vi "subvi_calculate_sizes.vi"(0 "Metadata":T7, 1 "font settings":T5={"Font Name:"="Arial", "Size"=12, "Strikeout?"=FALSE, "Italic?"=FALSE, "Underline?"=FALSE, "Outline?"=FALSE, "Shadow?"=FALSE, "Bold?"=FALSE}, 2 "Color settings":T6={"Background color"=0, "Information color"=16777215}, 3 "Spacing":T3, 4 "loaded picture":picture) -> (5 "modified pictures":picture)   [LabVIEW 2016]
uses:
  cluster_metadata.ctl
  cluster_colorsettings.ctl
  cluster_spacing.ctl
  cluster_background.ctl
panel:
  in  "Dimensions":T1
  in  "Coordinates":T2
  # "x and y are the distance between the\nlower left corner of the background box and the\nlower left corner of the bar"
  # "x and y are the distance between the\nlower left corner of the image and the\nlower left corner of the box"
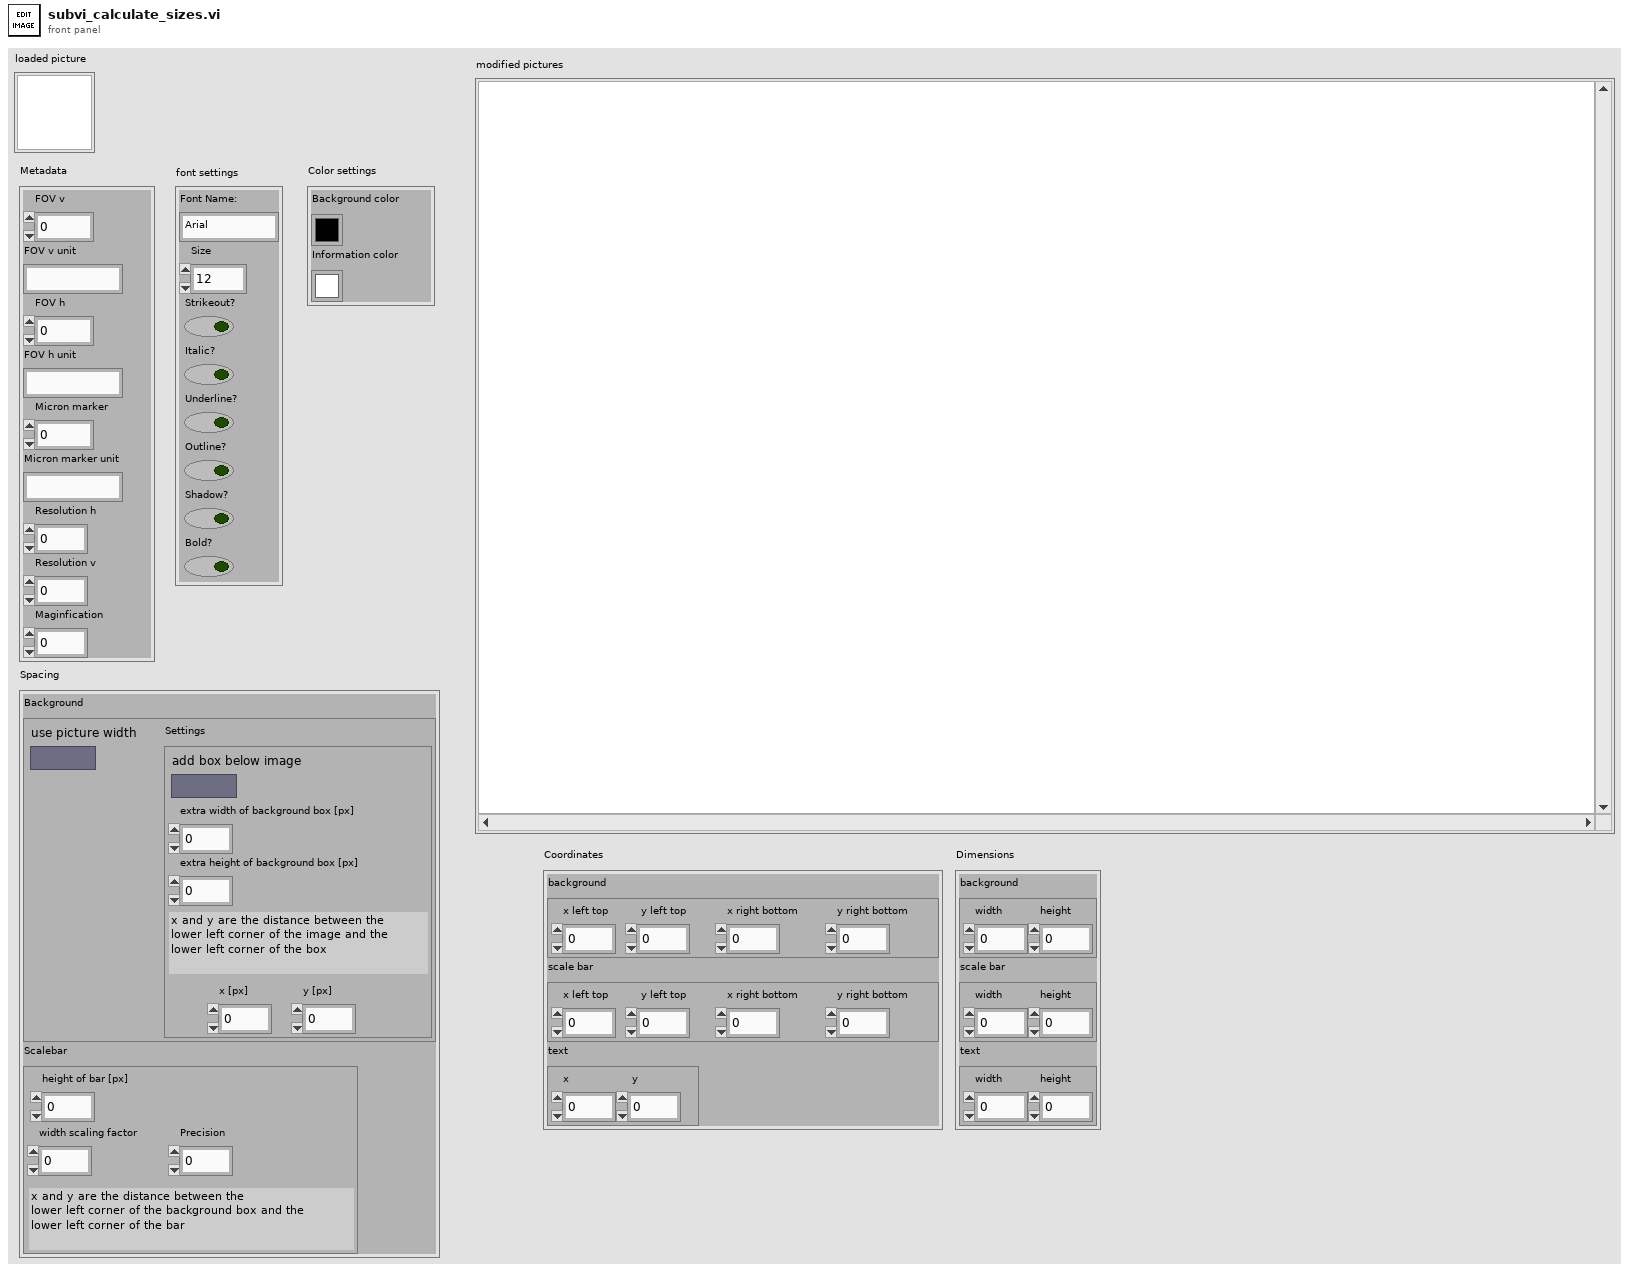
[diagram p1: front panel]
types:
  T1 = cluster{"background":cluster{"width":dbl, "height":dbl}, "scale bar":cluster{"width":dbl, "height":dbl}, "text":cluster{"width":dbl, "height":dbl}}
  T2 = cluster{"background":cluster{"x left top":dbl, "y left top":dbl, "x right bottom":dbl, "y right bottom":dbl}, "scale bar":cluster{"x left top":dbl, "y left top":dbl, "x right bottom":dbl, "y right bottom":dbl}, "text":cluster{"x ":dbl, "y":dbl}}
  T3 = typedef "cluster_spacing.ctl" = cluster{"Background":T4, "Scalebar":cluster{"height of bar [px]":dbl, "width scaling factor":dbl, "Precision":i16}}
  T4 = typedef "cluster_background.ctl" = cluster{"use picture width":bool, "Settings":cluster{"add box below image":bool, "extra width background":i16, "extra height background":i16, "x [px]":dbl, "y [px]":dbl}}
  T5 = cluster{"Font Name:":string, "Size":i16, "Strikeout?":bool, "Italic?":bool, "Underline?":bool, "Outline?":bool, "Shadow?":bool, "Bold?":bool}
  T6 = typedef "cluster_colorsettings.ctl" = cluster{"Background color":u32, "Information color":u32}
  T7 = typedef "cluster_metadata.ctl" = cluster{"FOV v":dbl, "FOV v unit":string, "FOV h":dbl, "FOV h unit":string, "Micron marker":dbl, "Micron marker unit":string, "Resolution h":i32, "Resolution v":i32, "Maginfication":i32}
  T8 = cluster{"horizontal":enum16{"left", "center", "right"}, "vertical":enum16{"top", "center", "bottom"}}
  T9 = enum16{"User-specified Font", "Application Font", "System Font", "Dialog Font"}
  T10 = cluster{"left":i16, "top":i16, "right":i16, "bottom":i16}
  T11 = cluster{"x left top":dbl, "y left top":dbl, "x right bottom":dbl, "y right bottom":dbl}
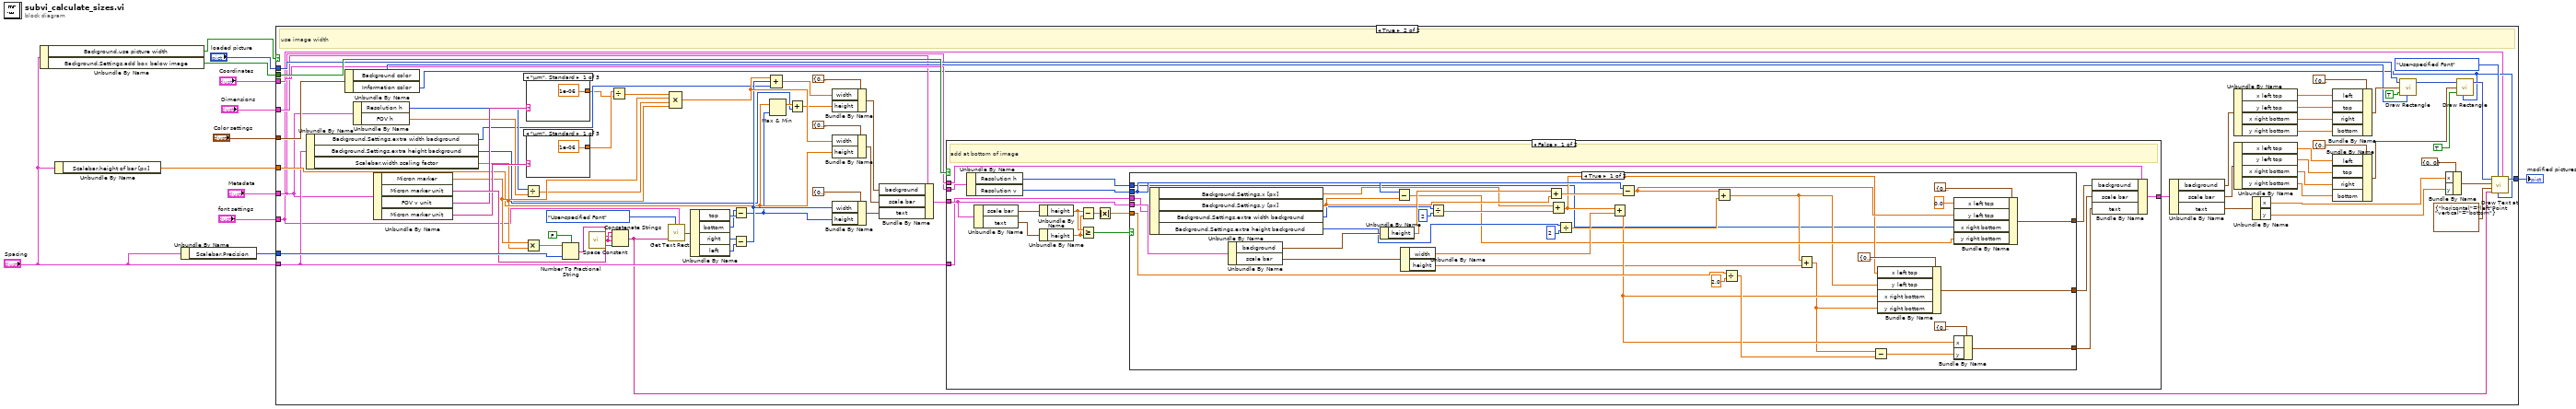
[diagram p0: block diagram]
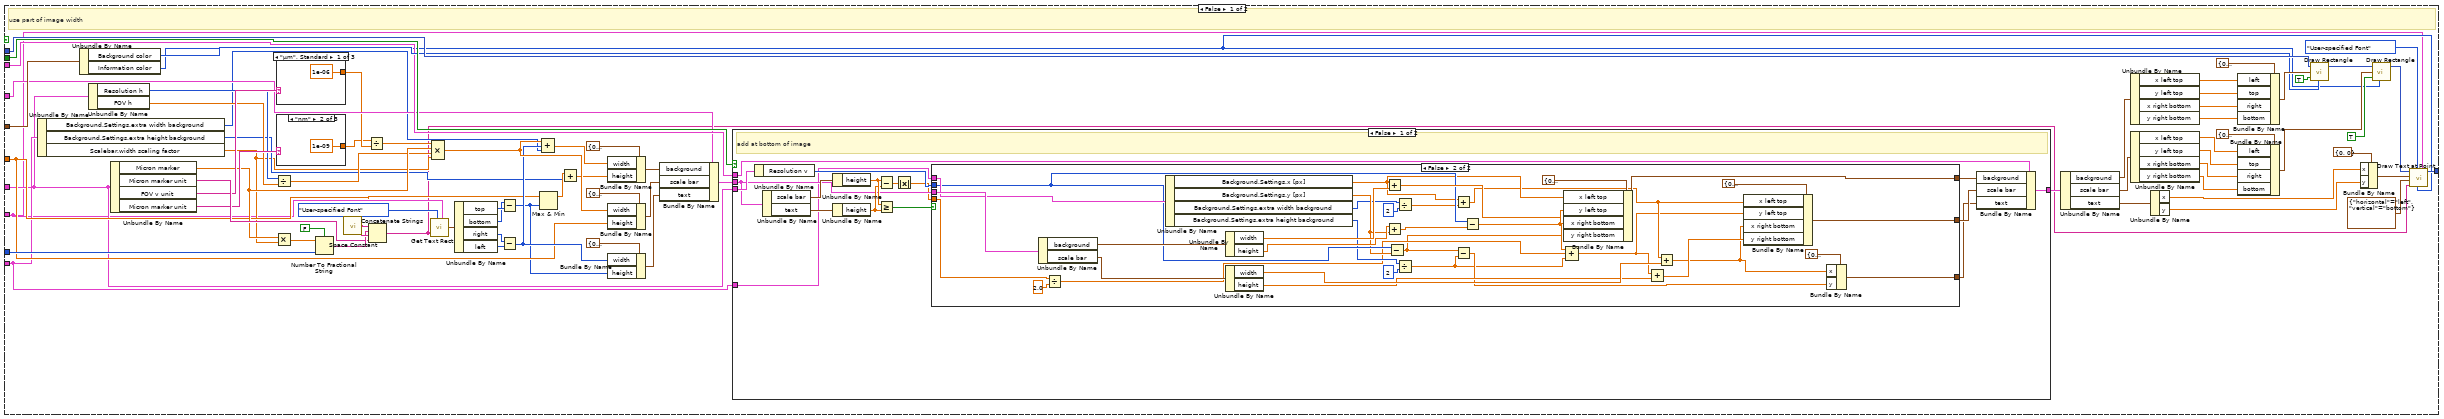
[diagram p2: hidden frame]
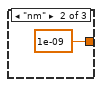
[diagram p3: hidden frame]
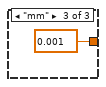
[diagram p4: hidden frame]
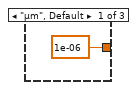
[diagram p5: hidden frame]
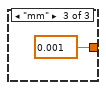
[diagram p6: hidden frame]
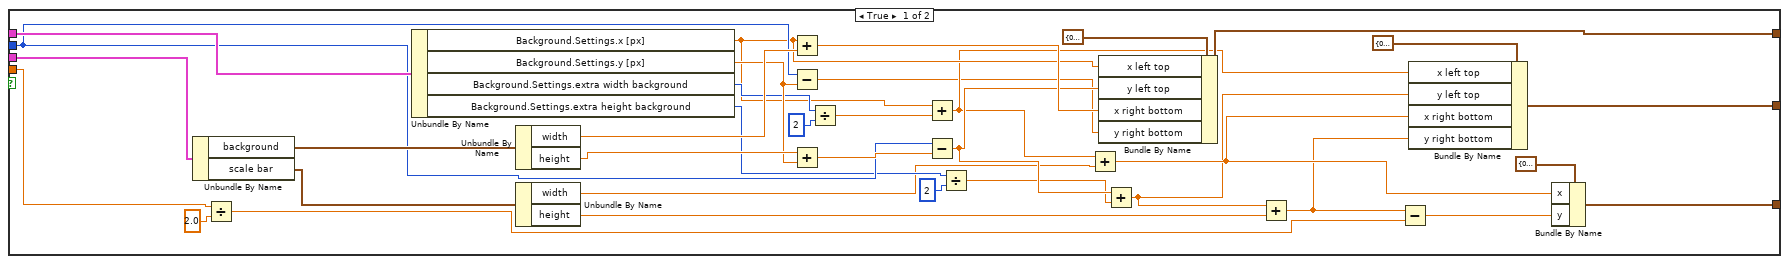
[diagram p7: hidden frame]
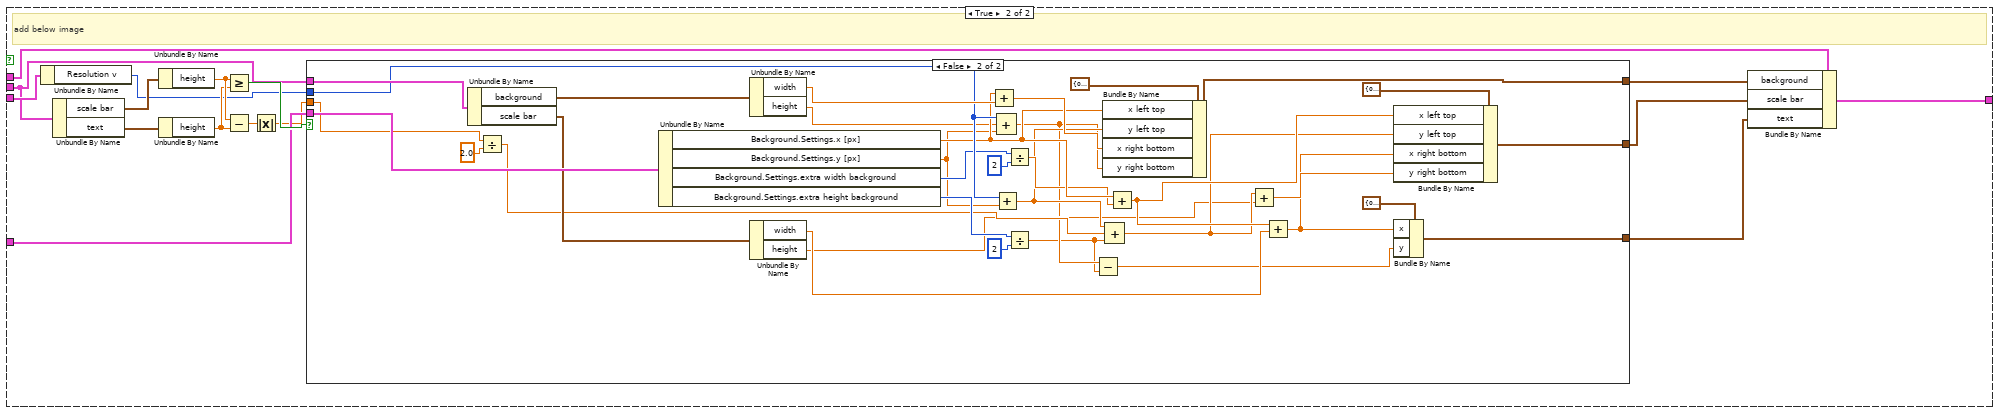
[diagram p8: hidden frame]
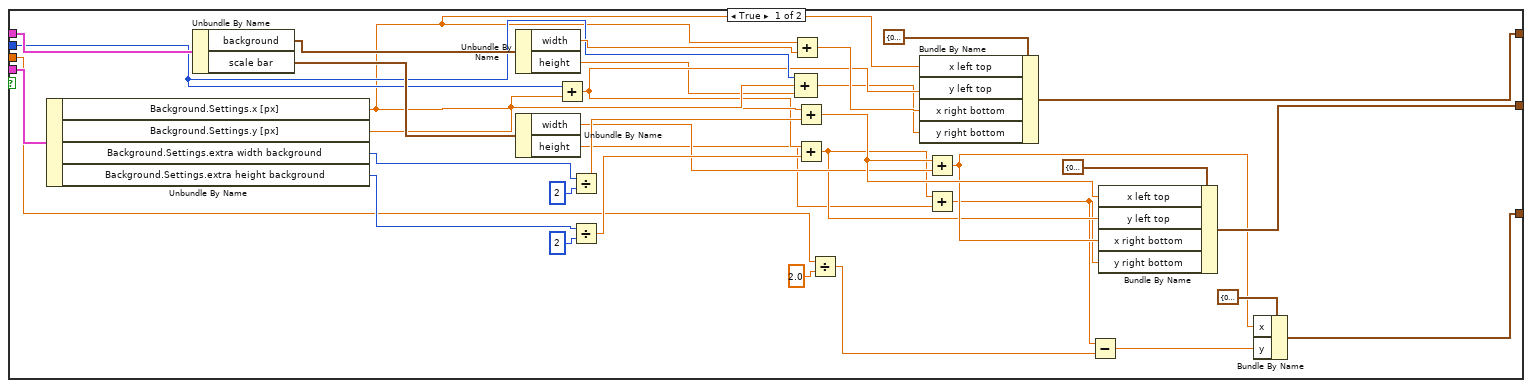
[diagram p9: hidden frame]
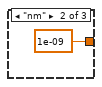
[diagram p10: hidden frame]
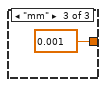
[diagram p11: hidden frame]
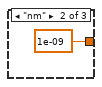
[diagram p12: hidden frame]
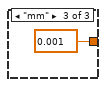
[diagram p13: hidden frame]
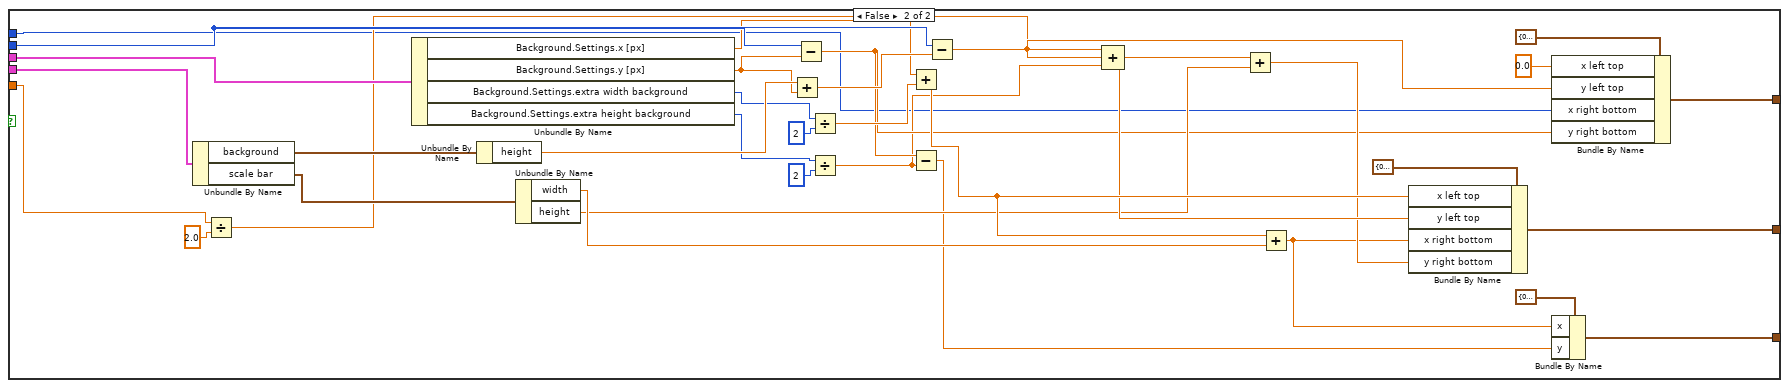
[diagram p14: hidden frame]
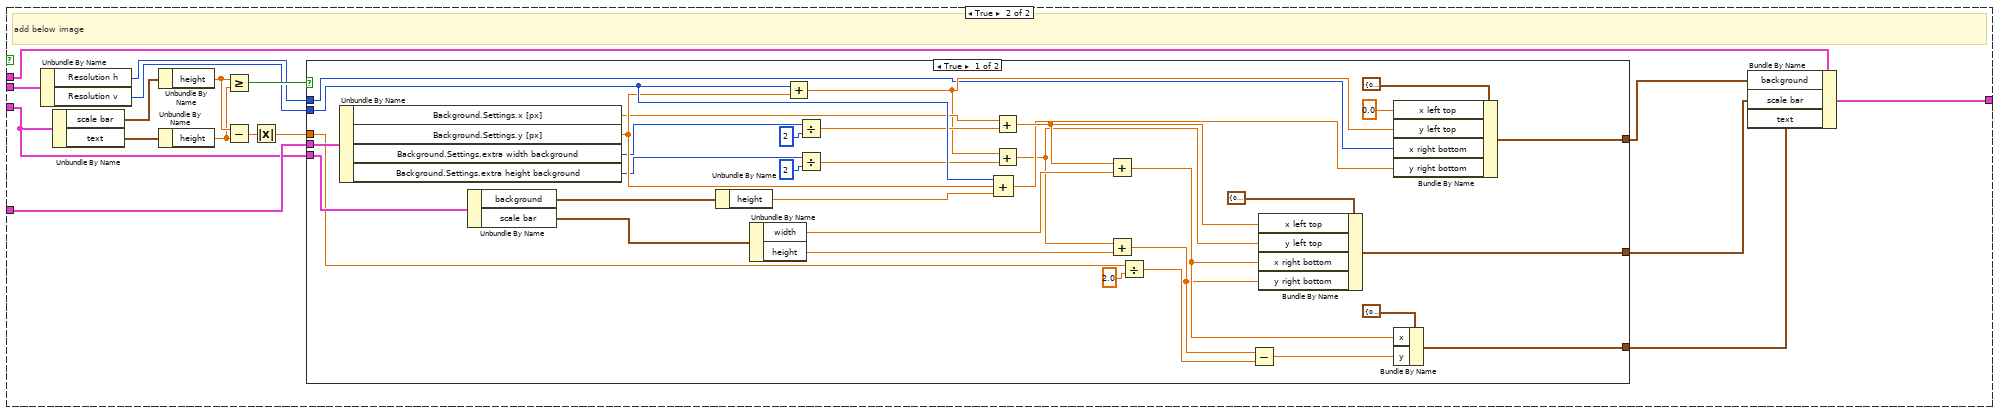
[diagram p15: hidden frame]
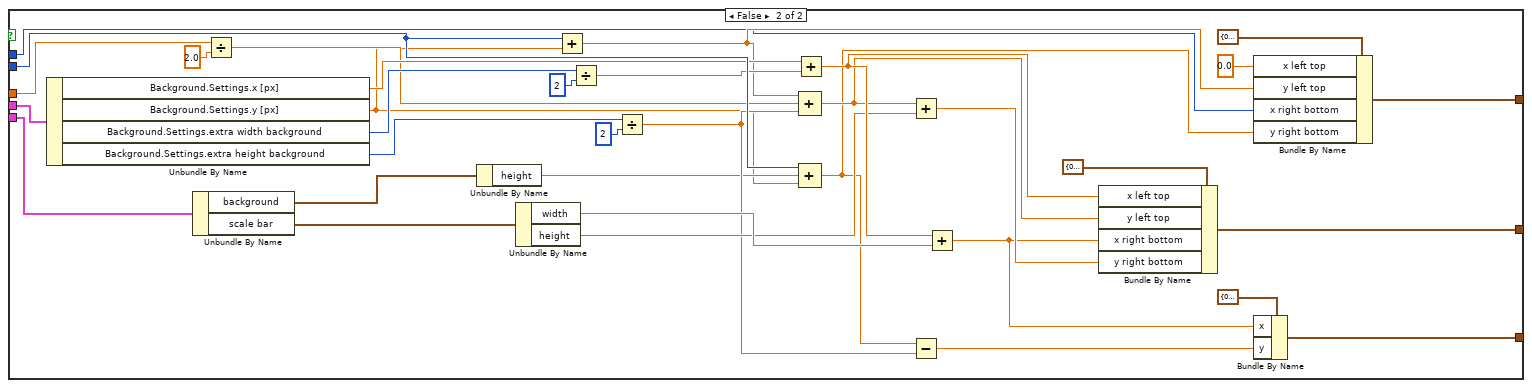
[diagram p16: hidden frame]
diagram:
  n1 = Unbundle By Name("Spacing") -> ("Background.use picture width"=w12:bool, "Background.Settings.add box below image"=w10:bool)
  n2 = Unbundle By Name("Spacing") -> ("Scalebar.height of bar [px]"=w4:dbl)
  n3 = Unbundle By Name("Spacing") -> ("Scalebar.Precision"=w1:i16)
  n4 = case "Case-Struktur" shown="True" w12 {
    tunnel: "loaded picture" -> [w75 w327]
    tunnel: w10 -> [w88 w340]
    tunnel: "Spacing" -> [w37 w289]
    tunnel: "Metadata" -> [w36 w288]
    tunnel: "font settings" -> [w19 w271]
    tunnel: w1 -> [w67 w319]
    tunnel: "Color settings" -> [w74 w326]
    tunnel: [w76 w328] -> w3
    tunnel: "Coordinates" -> [w55 w307]
    tunnel: "Dimensions" -> [w54 w306]
    tunnel: w4 -> [w40 w292]
    frame False {
      # "use part of image width"
      n5 = Unbundle By Name(w37) -> ("Background.Settings.extra width background"=w44:i16, "Background.Settings.extra height background"=w41:i16, "Scalebar.width scaling factor"=w35:dbl)
      n6 = Unbundle By Name(w74) -> ("Background color"=w73:u32, "Information color"=w20:u32)
      n7 = Unbundle By Name(w36) -> ("Resolution h"=w57:i32, "FOV h"=w56:dbl)
      n8 = Unbundle By Name(w36) -> ("Micron marker"=w59:dbl, "Micron marker unit"=w65:string, "FOV v unit"=w62:string, "Micron marker unit"=w61:string)
      n9 = Divide(x=w57, y=w56) -> (x/y=w58:dbl)
      n10 = Multiply(x=w59, y=w35) -> (x*y=w66:dbl)
      n11 = case shown="\"µm\", Standard" w62 {
        tunnel: [1e-06 1e-09 0.001] -> w14
        frame "µm", Default {
        }
        frame "nm" {
        }
        frame "mm" {
        }
      }
      n12 = case shown="\"nm\"" w61 {
        tunnel: [1e-06 1e-09 0.001] -> w13
        frame "µm", Default {
        }
        frame "nm" {
        }
        frame "mm" {
        }
      }
      n13 = Number To Fractional String(use system decimal point (T)=FALSE ("Systemdezimalzeichen verwenden (T)"), number=w66, precision (6)=w67) -> (F-format string=w70:string)  [unwired: 1 in]
      n14 = call <vilib>:"Space Constant.vi"() -> ("String"=w71:string)
      n15 = Divide(x=w13, y=w14) -> (x/y=w60:dbl)
      n16 = Concatenate Strings(w71, w70, w71, w65) -> (w18:string)
      n17 = call <vilib>:"Get Text Rect.vi"("desired font(Application)"=T9."User-specified Font", "text"=w18, "[user-specified font]"=w19) -> ("rect"=w72:T10)  [unwired: 6 in]
      n18 = Compound Arithmetic op=MULTIPLY(w60, w59, w58, w35) -> (w46:dbl)
      n19 = Unbundle By Name(w72) -> ("top"=w17:i16, "bottom"=w16:i16, "right"=w64:i16, "left"=w63:i16)
      n20 = Subtract(x=w16, y=w17) -> (x-y=w39:i16)
      n21 = Subtract(x=w64, y=w63) -> (x-y=w45:i16)
      n22 = Max & Min(x=w40, y=w39) -> (max(x,y)=w42:dbl)  [unwired: 1 out]
      n23 = Compound Arithmetic op=ADD(w46, w45, w44) -> (w48:dbl)
      n24 = Add(x=w42, y=w41) -> (x+y=w43:dbl)
      n25 = Bundle By Name(cluster=cluster{"width":dbl, "height":dbl} {"width"=0.0, "height"=0.0} ("text"), "width"=w48, "height"=w43) -> (w47:cluster{"width":dbl, "height":dbl})
      n26 = Bundle By Name(cluster=cluster{"width":dbl, "height":dbl} {"width"=0.0, "height"=0.0} ("text"), "width"=w46, "height"=w40) -> (w50:cluster{"width":dbl, "height":dbl})
      n27 = Bundle By Name(cluster=cluster{"width":dbl, "height":dbl} {"width"=0.0, "height"=0.0} ("text"), "width"=w45, "height"=w39) -> (w52:cluster{"width":dbl, "height":dbl})
      n28 = Bundle By Name(cluster=w54, "background"=w47, "scale bar"=w50, "text"=w52) -> (w38:T1)
      n29 = case shown="False" w88 {
        tunnel: w55 -> [w110 w196]
        tunnel: [w109 w195] -> w34
        tunnel: w38 -> [w101 w186]
        tunnel: w37 -> [w100 w187]
        tunnel: w36 -> [w108 w194]
        frame False {
          # "add at bottom of image"
          n30 = Unbundle By Name(w108) -> ("Resolution v"=w102:i32)
          n31 = Unbundle By Name(w101) -> ("scale bar"=w107:cluster{"width":dbl, "height":dbl}, "text"=w106:cluster{"width":dbl, "height":dbl})
          n32 = Unbundle By Name(w107) -> ("height"=w105:dbl)
          n33 = Unbundle By Name(w106) -> ("height"=w104:dbl)
          n34 = Subtract(x=w105, y=w104) -> (x-y=w103:dbl)
          n35 = Greater Or Equal?(x=w105, y=w104) -> (x >= y?=w98:bool)
          n36 = Absolute Value(x=w103) -> (abs(x)=w99:dbl)
          n37 = case shown="False" w98 {
            tunnel: [w144 w179] -> w96
            tunnel: w100 -> [w138 w173]
            tunnel: w101 -> [w143 w178]
            tunnel: [w141 w176] -> w95
            tunnel: w99 -> [w116 w159]
            tunnel: [w139 w174] -> w97
            tunnel: w102 -> [w131 w166]
            frame True {
              n38 = Unbundle By Name(w143) -> ("background"=w136:cluster{"width":dbl, "height":dbl}, "scale bar"=w137:cluster{"width":dbl, "height":dbl})
              n39 = Divide(x=w116, y=2.0) -> (x/y=w117:dbl)
              n40 = Unbundle By Name(w138) -> ("Background.Settings.x [px]"=w125:dbl, "Background.Settings.y [px]"=w130:dbl, "Background.Settings.extra width background"=w129:i16, "Background.Settings.extra height background"=w126:i16)
              n41 = Unbundle By Name(w136) -> ("width"=w132:dbl, "height"=w134:dbl)
              n42 = Unbundle By Name(w137) -> ("width"=w120:dbl, "height"=w112:dbl)
              n43 = Add(x=w125, y=w132) -> (x+y=w133:dbl)
              n44 = Subtract(x=w131, y=w130) -> (x-y=w119:dbl)
              n45 = Add(x=w134, y=w130) -> (x+y=w135:dbl)
              n46 = Divide(x=w129, y=i16 2) -> (x/y=w124:dbl)
              n47 = Add(x=w125, y=w124) -> (x+y=w121:dbl)
              n48 = Subtract(x=w131, y=w135) -> (x-y=w123:dbl)
              n49 = Divide(x=w126, y=i16 2) -> (x/y=w122:dbl)
              n50 = Add(x=w121, y=w120) -> (x+y=w114:dbl)
              n51 = Bundle By Name(cluster=T11 {"x left top"=0.0, "y left top"=0.0, "x right bottom"=0.0, "y right bottom"=0.0} ("background"), "x left top"=w125, "y left top"=w123, "x right bottom"=w133, "y right bottom"=w119) -> (w139:T11)
              n52 = Add(x=w123, y=w122) -> (x+y=w113:dbl)
              n53 = Add(x=w113, y=w112) -> (x+y=w111:dbl)
              n54 = Subtract(x=w111, y=w117) -> (x-y=w115:dbl)
              n55 = Bundle By Name(cluster=T11 {"x left top"=0.0, "y left top"=0.0, "x right bottom"=0.0, "y right bottom"=0.0} ("background"), "x left top"=w121, "y left top"=w113, "x right bottom"=w114, "y right bottom"=w111) -> (w144:T11)
              n56 = Bundle By Name(cluster=cluster{"x ":dbl, "y":dbl} {"x "=0.0, "y"=0.0} ("text"), "x"=w114, "y"=w115) -> (w141:cluster{"x ":dbl, "y":dbl})
            }
            frame False {
              n57 = Unbundle By Name(w178) -> ("background"=w171:cluster{"width":dbl, "height":dbl}, "scale bar"=w172:cluster{"width":dbl, "height":dbl})
              n58 = Divide(x=w159, y=2.0) -> (x/y=w153:dbl)
              n59 = Unbundle By Name(w173) -> ("Background.Settings.x [px]"=w158:dbl, "Background.Settings.y [px]"=w165:dbl, "Background.Settings.extra width background"=w164:i16, "Background.Settings.extra height background"=w161:i16)
              n60 = Unbundle By Name(w171) -> ("width"=w167:dbl, "height"=w169:dbl)
              n61 = Unbundle By Name(w172) -> ("width"=w155:dbl, "height"=w150:dbl)
              n62 = Add(x=w158, y=w167) -> (x+y=w168:dbl)
              n63 = Add(x=w169, y=w165) -> (x+y=w170:dbl)
              n64 = Subtract(x=w166, y=w165) -> (x-y=w147:dbl)
              n65 = Divide(x=w164, y=i16 2) -> (x/y=w157:dbl)
              n66 = Divide(x=w161, y=i16 2) -> (x/y=w146:dbl)
              n67 = Add(x=w158, y=w157) -> (x+y=w156:dbl)
              n68 = Subtract(x=w147, y=w146) -> (x-y=w148:dbl)
              n69 = Subtract(x=w166, y=w170) -> (x-y=w154:dbl)
              n70 = Bundle By Name(cluster=T11 {"x left top"=0.0, "y left top"=0.0, "x right bottom"=0.0, "y right bottom"=0.0} ("background"), "x left top"=w158, "y left top"=w154, "x right bottom"=w168, "y right bottom"=w147) -> (w174:T11)
              n71 = Compound Arithmetic op=ADD(w154, w153, w146) -> (w152:dbl)
              n72 = Add(x=w152, y=w150) -> (x+y=w151:dbl)
              n73 = Add(x=w156, y=w155) -> (x+y=w149:dbl)
              n74 = Bundle By Name(cluster=T11 {"x left top"=0.0, "y left top"=0.0, "x right bottom"=0.0, "y right bottom"=0.0} ("background"), "x left top"=w156, "y left top"=w152, "x right bottom"=w149, "y right bottom"=w151) -> (w179:T11)
              n75 = Bundle By Name(cluster=cluster{"x ":dbl, "y":dbl} {"x "=0.0, "y"=0.0} ("text"), "x"=w149, "y"=w148) -> (w176:cluster{"x ":dbl, "y":dbl})
            }
          }
          n76 = Bundle By Name(cluster=w110, "background"=w97, "scale bar"=w96, "text"=w95) -> (w109:T2)
        }
        frame True {
          # "add below image"
          n77 = Unbundle By Name(w194) -> ("Resolution v"=w185:i32)
          n78 = Unbundle By Name(w186) -> ("scale bar"=w193:cluster{"width":dbl, "height":dbl}, "text"=w192:cluster{"width":dbl, "height":dbl})
          n79 = Unbundle By Name(w193) -> ("height"=w191:dbl)
          n80 = Unbundle By Name(w192) -> ("height"=w190:dbl)
          n81 = Greater Or Equal?(x=w191, y=w190) -> (x >= y?=w188:bool)
          n82 = Subtract(x=w191, y=w190) -> (x-y=w189:dbl)
          n83 = Absolute Value(x=w189) -> (abs(x)=w184:dbl)
          n84 = case shown="False" w188 {
            tunnel: [w229 w263] -> w182
            tunnel: w187 -> [w223 w257]
            tunnel: w186 -> [w228 w262]
            tunnel: [w226 w260] -> w183
            tunnel: w184 -> [w203 w246]
            tunnel: [w224 w258] -> w181
            tunnel: w185 -> [w218 w252]
            frame True {
              n85 = Unbundle By Name(w223) -> ("Background.Settings.x [px]"=w212:dbl, "Background.Settings.y [px]"=w217:dbl, "Background.Settings.extra width background"=w216:i16, "Background.Settings.extra height background"=w213:i16)
              n86 = Unbundle By Name(w228) -> ("background"=w221:cluster{"width":dbl, "height":dbl}, "scale bar"=w222:cluster{"width":dbl, "height":dbl})
              n87 = Unbundle By Name(w221) -> ("width"=w219:dbl, "height"=w197:dbl)
              n88 = Unbundle By Name(w222) -> ("width"=w207:dbl, "height"=w199:dbl)
              n89 = Add(x=w218, y=w217) -> (x+y=w210:dbl)
              n90 = Divide(x=w216, y=i16 2) -> (x/y=w211:dbl)
              n91 = Divide(x=w213, y=i16 2) -> (x/y=w209:dbl)
              n92 = Add(x=w212, y=w219) -> (x+y=w220:dbl)
              n93 = Compound Arithmetic op=ADD(w218, w217, w197) -> (w206:dbl)
              n94 = Add(x=w212, y=w211) -> (x+y=w208:dbl)
              n95 = Add(x=w210, y=w209) -> (x+y=w200:dbl)
              n96 = Divide(x=w203, y=2.0) -> (x/y=w204:dbl)
              n97 = Bundle By Name(cluster=T11 {"x left top"=0.0, "y left top"=0.0, "x right bottom"=0.0, "y right bottom"=0.0} ("background"), "x left top"=w212, "y left top"=w210, "x right bottom"=w220, "y right bottom"=w206) -> (w224:T11)
              n98 = Add(x=w208, y=w207) -> (x+y=w201:dbl)
              n99 = Add(x=w200, y=w199) -> (x+y=w198:dbl)
              n100 = Subtract(x=w198, y=w204) -> (x-y=w202:dbl)
              n101 = Bundle By Name(cluster=T11 {"x left top"=0.0, "y left top"=0.0, "x right bottom"=0.0, "y right bottom"=0.0} ("background"), "x left top"=w208, "y left top"=w200, "x right bottom"=w201, "y right bottom"=w198) -> (w229:T11)
              n102 = Bundle By Name(cluster=cluster{"x ":dbl, "y":dbl} {"x "=0.0, "y"=0.0} ("text"), "x"=w201, "y"=w202) -> (w226:cluster{"x ":dbl, "y":dbl})
            }
            frame False {
              n103 = Unbundle By Name(w262) -> ("background"=w255:cluster{"width":dbl, "height":dbl}, "scale bar"=w256:cluster{"width":dbl, "height":dbl})
              n104 = Divide(x=w246, y=2.0) -> (x/y=w240:dbl)
              n105 = Unbundle By Name(w257) -> ("Background.Settings.x [px]"=w245:dbl, "Background.Settings.y [px]"=w231:dbl, "Background.Settings.extra width background"=w251:i16, "Background.Settings.extra height background"=w248:i16)
              n106 = Unbundle By Name(w255) -> ("width"=w253:dbl, "height"=w232:dbl)
              n107 = Unbundle By Name(w256) -> ("width"=w242:dbl, "height"=w237:dbl)
              n108 = Add(x=w245, y=w253) -> (x+y=w254:dbl)
              n109 = Add(x=w252, y=w231) -> (x+y=w241:dbl)
              n110 = Compound Arithmetic op=ADD(w252, w232, w231) -> (w234:dbl)
              n111 = Divide(x=w251, y=i16 2) -> (x/y=w244:dbl)
              n112 = Divide(x=w248, y=i16 2) -> (x/y=w233:dbl)
              n113 = Subtract(x=w234, y=w233) -> (x-y=w235:dbl)
              n114 = Bundle By Name(cluster=T11 {"x left top"=0.0, "y left top"=0.0, "x right bottom"=0.0, "y right bottom"=0.0} ("background"), "x left top"=w245, "y left top"=w241, "x right bottom"=w254, "y right bottom"=w234) -> (w258:T11)
              n115 = Compound Arithmetic op=ADD(w241, w240, w233) -> (w239:dbl)
              n116 = Add(x=w245, y=w244) -> (x+y=w243:dbl)
              n117 = Add(x=w239, y=w237) -> (x+y=w238:dbl)
              n118 = Add(x=w243, y=w242) -> (x+y=w236:dbl)
              n119 = Bundle By Name(cluster=T11 {"x left top"=0.0, "y left top"=0.0, "x right bottom"=0.0, "y right bottom"=0.0} ("background"), "x left top"=w243, "y left top"=w239, "x right bottom"=w236, "y right bottom"=w238) -> (w263:T11)
              n120 = Bundle By Name(cluster=cluster{"x ":dbl, "y":dbl} {"x "=0.0, "y"=0.0} ("text"), "x"=w236, "y"=w235) -> (w260:cluster{"x ":dbl, "y":dbl})
            }
          }
          n121 = Bundle By Name(cluster=w196, "background"=w181, "scale bar"=w182, "text"=w183) -> (w195:T2)
        }
      }
      n122 = Unbundle By Name(w34) -> ("background"=w33:T11, "scale bar"=w28:T11, "text"=w23:cluster{"x ":dbl, "y":dbl})
      n123 = Unbundle By Name(w33) -> ("x left top"=w32:dbl, "y left top"=w31:dbl, "x right bottom"=w30:dbl, "y right bottom"=w29:dbl)
      n124 = Unbundle By Name(w28) -> ("x left top"=w27:dbl, "y left top"=w26:dbl, "x right bottom"=w25:dbl, "y right bottom"=w24:dbl)
      n125 = Unbundle By Name(w23) -> ("x"=w22:dbl, "y"=w21:dbl)
      n126 = Bundle By Name(cluster=T10 {"left"=0, "top"=0, "right"=0, "bottom"=0} ("rect"), "left"=w32, "top"=w31, "right"=w30, "bottom"=w29) -> (w86:T10)
      n127 = Bundle By Name(cluster=T10 {"left"=0, "top"=0, "right"=0, "bottom"=0} ("rect"), "left"=w27, "top"=w26, "right"=w25, "bottom"=w24) -> (w84:T10)
      n128 = call <vilib>:"Draw Rectangle.vi"("picture"=w75, "rect"=w86, "fill?(F)"=TRUE, "color(black)"=w73) -> ("new picture"=w81:picture)  [unwired: 5 in]
      n129 = Bundle By Name(cluster=cluster{"x":i16, "y":i16} {"x"=0, "y"=0} ("origin"), "x"=w22, "y"=w21) -> (w79:cluster{"x":i16, "y":i16})
      n130 = call <vilib>:"Draw Rectangle.vi"("picture"=w81, "rect"=w84, "fill?(F)"=TRUE, "color(black)"=w20) -> ("new picture"=w77:picture)  [unwired: 5 in]
      n131 = call <vilib>:"Draw Text at Point.vi"("[user-specified font]"=w19, "text color(black)"=w20, "desired font(Application)"=T9."User-specified Font", "text"=w18, "alignment(left, top)"=T8 {"horizontal"=enum."left", "vertical"=enum."bottom"}, "origin"=w79, "picture"=w77) -> ("new picture"=w76:picture)  [unwired: 3 in, 1 out]
    }
    frame True {
      # "use image width"
      n132 = Unbundle By Name(w289) -> ("Background.Settings.extra width background"=w296:i16, "Background.Settings.extra height background"=w293:i16, "Scalebar.width scaling factor"=w287:dbl)
      n133 = Unbundle By Name(w326) -> ("Background color"=w325:u32, "Information color"=w272:u32)
      n134 = Unbundle By Name(w288) -> ("Resolution h"=w309:i32, "FOV h"=w308:dbl)
      n135 = Unbundle By Name(w288) -> ("Micron marker"=w311:dbl, "Micron marker unit"=w317:string, "FOV v unit"=w314:string, "Micron marker unit"=w313:string)
      n136 = Divide(x=w309, y=w308) -> (x/y=w310:dbl)
      n137 = Multiply(x=w311, y=w287) -> (x*y=w318:dbl)
      n138 = case shown="\"µm\", Standard" w314 {
        tunnel: [1e-06 1e-09 0.001] -> w265
        frame "µm", Default {
        }
        frame "nm" {
        }
        frame "mm" {
        }
      }
      n139 = case shown="\"µm\", Standard" w313 {
        tunnel: [1e-06 1e-09 0.001] -> w266
        frame "µm", Default {
        }
        frame "nm" {
        }
        frame "mm" {
        }
      }
      n140 = Number To Fractional String(use system decimal point (T)=FALSE ("Systemdezimalzeichen verwenden (T)"), number=w318, precision (6)=w319) -> (F-format string=w322:string)  [unwired: 1 in]
      n141 = call <vilib>:"Space Constant.vi"() -> ("String"=w323:string)
      n142 = Divide(x=w266, y=w265) -> (x/y=w312:dbl)
      n143 = Concatenate Strings(w323, w322, w323, w317) -> (w270:string)
      n144 = call <vilib>:"Get Text Rect.vi"("desired font(Application)"=T9."User-specified Font", "text"=w270, "[user-specified font]"=w271) -> ("rect"=w324:T10)  [unwired: 6 in]
      n145 = Compound Arithmetic op=MULTIPLY(w312, w311, w310, w287) -> (w298:dbl)
      n146 = Unbundle By Name(w324) -> ("top"=w269:i16, "bottom"=w268:i16, "right"=w316:i16, "left"=w315:i16)
      n147 = Subtract(x=w268, y=w269) -> (x-y=w291:i16)
      n148 = Subtract(x=w316, y=w315) -> (x-y=w297:i16)
      n149 = Max & Min(x=w292, y=w291) -> (max(x,y)=w294:dbl)  [unwired: 1 out]
      n150 = Compound Arithmetic op=ADD(w298, w297, w296) -> (w300:dbl)
      n151 = Add(x=w294, y=w293) -> (x+y=w295:dbl)
      n152 = Bundle By Name(cluster=cluster{"width":dbl, "height":dbl} {"width"=0.0, "height"=0.0} ("text"), "width"=w300, "height"=w295) -> (w299:cluster{"width":dbl, "height":dbl})
      n153 = Bundle By Name(cluster=cluster{"width":dbl, "height":dbl} {"width"=0.0, "height"=0.0} ("text"), "width"=w298, "height"=w292) -> (w302:cluster{"width":dbl, "height":dbl})
      n154 = Bundle By Name(cluster=cluster{"width":dbl, "height":dbl} {"width"=0.0, "height"=0.0} ("text"), "width"=w297, "height"=w291) -> (w304:cluster{"width":dbl, "height":dbl})
      n155 = Bundle By Name(cluster=w306, "background"=w299, "scale bar"=w302, "text"=w304) -> (w290:T1)
      n156 = case shown="False" w340 {
        tunnel: w307 -> [w363 w450]
        tunnel: [w362 w449] -> w286
        tunnel: w290 -> [w354 w440]
        tunnel: w289 -> [w353 w441]
        tunnel: w288 -> [w361 w448]
        frame False {
          # "add at bottom of image"
          n157 = Unbundle By Name(w361) -> ("Resolution h"=w347:i32, "Resolution v"=w355:i32)
          n158 = Unbundle By Name(w354) -> ("scale bar"=w360:cluster{"width":dbl, "height":dbl}, "text"=w359:cluster{"width":dbl, "height":dbl})
          n159 = Unbundle By Name(w360) -> ("height"=w358:dbl)
          n160 = Unbundle By Name(w359) -> ("height"=w357:dbl)
          n161 = Subtract(x=w358, y=w357) -> (x-y=w356:dbl)
          n162 = Greater Or Equal?(x=w358, y=w357) -> (x >= y?=w351:bool)
          n163 = Absolute Value(x=w356) -> (abs(x)=w352:dbl)
          n164 = case shown="True" w351 {
            tunnel: [w397 w432] -> w349
            tunnel: w353 -> [w391 w426]
            tunnel: w354 -> [w396 w431]
            tunnel: [w394 w429] -> w348
            tunnel: w352 -> [w371 w414]
            tunnel: [w392 w427] -> w350
            tunnel: w355 -> [w386 w421]
            tunnel: w347 -> [w365 w399]
            frame True {
              n165 = Unbundle By Name(w391) -> ("Background.Settings.x [px]"=w380:dbl, "Background.Settings.y [px]"=w385:dbl, "Background.Settings.extra width background"=w384:i16, "Background.Settings.extra height background"=w381:i16)
              n166 = Unbundle By Name(w396) -> ("background"=w389:cluster{"width":dbl, "height":dbl}, "scale bar"=w390:cluster{"width":dbl, "height":dbl})
              n167 = Unbundle By Name(w389) -> ("height"=w387:dbl)
              n168 = Subtract(x=w386, y=w385) -> (x-y=w374:dbl)
              n169 = Unbundle By Name(w390) -> ("width"=w375:dbl, "height"=w367:dbl)
              n170 = Divide(x=w384, y=i16 2) -> (x/y=w379:dbl)
              n171 = Add(x=w387, y=w385) -> (x+y=w388:dbl)
              n172 = Add(x=w380, y=w379) -> (x+y=w376:dbl)
              n173 = Divide(x=w381, y=i16 2) -> (x/y=w377:dbl)
              n174 = Add(x=w376, y=w375) -> (x+y=w369:dbl)
              n175 = Subtract(x=w386, y=w388) -> (x-y=w378:dbl)
              n176 = Add(x=w378, y=w377) -> (x+y=w368:dbl)
              n177 = Divide(x=w371, y=2.0) -> (x/y=w372:dbl)
              n178 = Add(x=w368, y=w367) -> (x+y=w366:dbl)
              n179 = Subtract(x=w366, y=w372) -> (x-y=w370:dbl)
              n180 = Bundle By Name(cluster=T11 {"x left top"=0.0, "y left top"=0.0, "x right bottom"=0.0, "y right bottom"=0.0} ("background"), "x left top"=w376, "y left top"=w368, "x right bottom"=w369, "y right bottom"=w366) -> (w397:T11)
              n181 = Bundle By Name(cluster=T11 {"x left top"=0.0, "y left top"=0.0, "x right bottom"=0.0, "y right bottom"=0.0} ("background"), "x left top"=0.0, "y left top"=w378, "x right bottom"=w365, "y right bottom"=w374) -> (w392:T11)
              n182 = Bundle By Name(cluster=cluster{"x ":dbl, "y":dbl} {"x "=0.0, "y"=0.0} ("text"), "x"=w369, "y"=w370) -> (w394:cluster{"x ":dbl, "y":dbl})
            }
            frame False {
              n183 = Unbundle By Name(w431) -> ("background"=w424:cluster{"width":dbl, "height":dbl}, "scale bar"=w425:cluster{"width":dbl, "height":dbl})
              n184 = Divide(x=w414, y=2.0) -> (x/y=w408:dbl)
              n185 = Unbundle By Name(w426) -> ("Background.Settings.x [px]"=w413:dbl, "Background.Settings.y [px]"=w420:dbl, "Background.Settings.extra width background"=w419:i16, "Background.Settings.extra height background"=w416:i16)
              n186 = Unbundle By Name(w424) -> ("height"=w422:dbl)
              n187 = Unbundle By Name(w425) -> ("width"=w410:dbl, "height"=w405:dbl)
              n188 = Add(x=w422, y=w420) -> (x+y=w423:dbl)
              n189 = Subtract(x=w421, y=w420) -> (x-y=w402:dbl)
              n190 = Divide(x=w419, y=i16 2) -> (x/y=w412:dbl)
              n191 = Divide(x=w416, y=i16 2) -> (x/y=w401:dbl)
              n192 = Add(x=w413, y=w412) -> (x+y=w411:dbl)
              n193 = Subtract(x=w402, y=w401) -> (x-y=w403:dbl)
              n194 = Subtract(x=w421, y=w423) -> (x-y=w409:dbl)
              n195 = Compound Arithmetic op=ADD(w409, w408, w401) -> (w407:dbl)
              n196 = Add(x=w407, y=w405) -> (x+y=w406:dbl)
              n197 = Add(x=w411, y=w410) -> (x+y=w404:dbl)
              n198 = Bundle By Name(cluster=T11 {"x left top"=0.0, "y left top"=0.0, "x right bottom"=0.0, "y right bottom"=0.0} ("background"), "x left top"=w411, "y left top"=w407, "x right bottom"=w404, "y right bottom"=w406) -> (w432:T11)
              n199 = Bundle By Name(cluster=T11 {"x left top"=0.0, "y left top"=0.0, "x right bottom"=0.0, "y right bottom"=0.0} ("background"), "x left top"=0.0, "y left top"=w409, "x right bottom"=w399, "y right bottom"=w402) -> (w427:T11)
              n200 = Bundle By Name(cluster=cluster{"x ":dbl, "y":dbl} {"x "=0.0, "y"=0.0} ("text"), "x"=w404, "y"=w403) -> (w429:cluster{"x ":dbl, "y":dbl})
            }
          }
          n201 = Bundle By Name(cluster=w363, "background"=w350, "scale bar"=w349, "text"=w348) -> (w362:T2)
        }
        frame True {
          # "add below image"
          n202 = Unbundle By Name(w448) -> ("Resolution h"=w434:i32, "Resolution v"=w439:i32)
          n203 = Unbundle By Name(w440) -> ("scale bar"=w447:cluster{"width":dbl, "height":dbl}, "text"=w446:cluster{"width":dbl, "height":dbl})
          n204 = Unbundle By Name(w447) -> ("height"=w445:dbl)
          n205 = Unbundle By Name(w446) -> ("height"=w444:dbl)
          n206 = Greater Or Equal?(x=w445, y=w444) -> (x >= y?=w442:bool)
          n207 = Subtract(x=w445, y=w444) -> (x-y=w443:dbl)
          n208 = Absolute Value(x=w443) -> (abs(x)=w438:dbl)
          n209 = case shown="True" w442 {
            tunnel: [w483 w517] -> w436
            tunnel: w441 -> [w477 w511]
            tunnel: w440 -> [w482 w516]
            tunnel: [w480 w514] -> w437
            tunnel: w438 -> [w459 w502]
            tunnel: [w478 w512] -> w435
            tunnel: w439 -> [w474 w508]
            tunnel: w434 -> [w451 w485]
            frame True {
              n210 = Unbundle By Name(w477) -> ("Background.Settings.x [px]"=w468:dbl, "Background.Settings.y [px]"=w473:dbl, "Background.Settings.extra width background"=w472:i16, "Background.Settings.extra height background"=w469:i16)
              n211 = Unbundle By Name(w482) -> ("background"=w475:cluster{"width":dbl, "height":dbl}, "scale bar"=w476:cluster{"width":dbl, "height":dbl})
              n212 = Unbundle By Name(w475) -> ("height"=w453:dbl)
              n213 = Unbundle By Name(w476) -> ("width"=w463:dbl, "height"=w455:dbl)
              n214 = Add(x=w474, y=w473) -> (x+y=w466:dbl)
              n215 = Divide(x=w472, y=i16 2) -> (x/y=w467:dbl)
              n216 = Divide(x=w469, y=i16 2) -> (x/y=w465:dbl)
              n217 = Compound Arithmetic op=ADD(w474, w473, w453) -> (w462:dbl)
              n218 = Add(x=w468, y=w467) -> (x+y=w464:dbl)
              n219 = Add(x=w466, y=w465) -> (x+y=w456:dbl)
              n220 = Add(x=w464, y=w463) -> (x+y=w457:dbl)
              n221 = Add(x=w456, y=w455) -> (x+y=w454:dbl)
              n222 = Divide(x=w459, y=2.0) -> (x/y=w460:dbl)
              n223 = Subtract(x=w454, y=w460) -> (x-y=w458:dbl)
              n224 = Bundle By Name(cluster=T11 {"x left top"=0.0, "y left top"=0.0, "x right bottom"=0.0, "y right bottom"=0.0} ("background"), "x left top"=w464, "y left top"=w456, "x right bottom"=w457, "y right bottom"=w454) -> (w483:T11)
              n225 = Bundle By Name(cluster=T11 {"x left top"=0.0, "y left top"=0.0, "x right bottom"=0.0, "y right bottom"=0.0} ("background"), "x left top"=0.0, "y left top"=w466, "x right bottom"=w451, "y right bottom"=w462) -> (w478:T11)
              n226 = Bundle By Name(cluster=cluster{"x ":dbl, "y":dbl} {"x "=0.0, "y"=0.0} ("text"), "x"=w457, "y"=w458) -> (w480:cluster{"x ":dbl, "y":dbl})
            }
            frame False {
              n227 = Unbundle By Name(w511) -> ("Background.Settings.x [px]"=w501:dbl, "Background.Settings.y [px]"=w487:dbl, "Background.Settings.extra width background"=w507:i16, "Background.Settings.extra height background"=w504:i16)
              n228 = Unbundle By Name(w516) -> ("background"=w509:cluster{"width":dbl, "height":dbl}, "scale bar"=w510:cluster{"width":dbl, "height":dbl})
              n229 = Divide(x=w502, y=2.0) -> (x/y=w496:dbl)
              n230 = Unbundle By Name(w509) -> ("height"=w488:dbl)
              n231 = Unbundle By Name(w510) -> ("width"=w498:dbl, "height"=w493:dbl)
              n232 = Add(x=w508, y=w487) -> (x+y=w497:dbl)
              n233 = Divide(x=w507, y=i16 2) -> (x/y=w500:dbl)
              n234 = Divide(x=w504, y=i16 2) -> (x/y=w489:dbl)
              n235 = Add(x=w501, y=w500) -> (x+y=w499:dbl)
              n236 = Compound Arithmetic op=ADD(w497, w496, w489) -> (w495:dbl)
              n237 = Compound Arithmetic op=ADD(w508, w488, w487) -> (w490:dbl)
              n238 = Add(x=w495, y=w493) -> (x+y=w494:dbl)
              n239 = Subtract(x=w490, y=w489) -> (x-y=w491:dbl)
              n240 = Add(x=w499, y=w498) -> (x+y=w492:dbl)
              n241 = Bundle By Name(cluster=T11 {"x left top"=0.0, "y left top"=0.0, "x right bottom"=0.0, "y right bottom"=0.0} ("background"), "x left top"=w499, "y left top"=w495, "x right bottom"=w492, "y right bottom"=w494) -> (w517:T11)
              n242 = Bundle By Name(cluster=T11 {"x left top"=0.0, "y left top"=0.0, "x right bottom"=0.0, "y right bottom"=0.0} ("background"), "x left top"=0.0, "y left top"=w497, "x right bottom"=w485, "y right bottom"=w490) -> (w512:T11)
              n243 = Bundle By Name(cluster=cluster{"x ":dbl, "y":dbl} {"x "=0.0, "y"=0.0} ("text"), "x"=w492, "y"=w491) -> (w514:cluster{"x ":dbl, "y":dbl})
            }
          }
          n244 = Bundle By Name(cluster=w450, "background"=w435, "scale bar"=w436, "text"=w437) -> (w449:T2)
        }
      }
      n245 = Unbundle By Name(w286) -> ("background"=w285:T11, "scale bar"=w280:T11, "text"=w275:cluster{"x ":dbl, "y":dbl})
      n246 = Unbundle By Name(w285) -> ("x left top"=w284:dbl, "y left top"=w283:dbl, "x right bottom"=w282:dbl, "y right bottom"=w281:dbl)
      n247 = Unbundle By Name(w280) -> ("x left top"=w279:dbl, "y left top"=w278:dbl, "x right bottom"=w277:dbl, "y right bottom"=w276:dbl)
      n248 = Unbundle By Name(w275) -> ("x"=w274:dbl, "y"=w273:dbl)
      n249 = Bundle By Name(cluster=T10 {"left"=0, "top"=0, "right"=0, "bottom"=0} ("rect"), "left"=w284, "top"=w283, "right"=w282, "bottom"=w281) -> (w338:T10)
      n250 = Bundle By Name(cluster=T10 {"left"=0, "top"=0, "right"=0, "bottom"=0} ("rect"), "left"=w279, "top"=w278, "right"=w277, "bottom"=w276) -> (w336:T10)
      n251 = call <vilib>:"Draw Rectangle.vi"("picture"=w327, "rect"=w338, "fill?(F)"=TRUE, "color(black)"=w325) -> ("new picture"=w333:picture)  [unwired: 5 in]
      n252 = Bundle By Name(cluster=cluster{"x":i16, "y":i16} {"x"=0, "y"=0} ("origin"), "x"=w274, "y"=w273) -> (w331:cluster{"x":i16, "y":i16})
      n253 = call <vilib>:"Draw Rectangle.vi"("picture"=w333, "rect"=w336, "fill?(F)"=TRUE, "color(black)"=w272) -> ("new picture"=w329:picture)  [unwired: 5 in]
      n254 = call <vilib>:"Draw Text at Point.vi"("[user-specified font]"=w271, "text color(black)"=w272, "desired font(Application)"=T9."User-specified Font", "text"=w270, "alignment(left, top)"=T8 {"horizontal"=enum."left", "vertical"=enum."bottom"}, "origin"=w331, "picture"=w329) -> ("new picture"=w328:picture)  [unwired: 3 in, 1 out]
    }
  }
  "modified pictures" <- w3
